vi "Handle Data Change.vi"(4 "Value":string, 6 "Combo Box Ref":refnum<vi>, 7 "Data in":path, 8 "error in (no error)":errorcluster, 9 "Run Mode?":bool, 10 "Indicator?":bool, 11 "Path Selector in":refnum<class "MGI Path Selector.lvclass">) -> (0 "error out":errorcluster, 3 "Path Selector out":refnum<class "MGI Path Selector.lvclass">, 5 "Data out":path)   [LabVIEW 2020, in "MGI Path Selector.lvclass"]
doc: "Take an action appropriate for the specified value of the combo box.\n\nAuthored by Shawn Walpole\nsupport@mooregoodideas.com\nwww.mooregoodideas.com\n\nCopyright (c) 2013, Moore Good Ideas, Inc.\n\nAll rights reserved.\n\nRedistribution and use in source and binary forms, with or without modification, are permitted provided that the following conditions are met:\n\n * Redistributions of source code must retain the above copyright notice, this list of conditions and the following disclaimer.\n * Redistributions in binary form must reproduce the above copyright notice, this list of conditions and the following disclaimer in the documentation and/or other materials provided with the distribution.\n * Neither the name of Moore Good Ideas, Inc. nor the names of its contributors may be used to endorse or promote products derived from this software without specific prior written permission.\n\nTHIS SOFTWARE IS PROVIDED BY THE COPYRIGHT HOLDERS AND CONTRIBUTORS \"AS IS\" AND ANY EXPRESS OR IMPLIED WARRANTIES, INCLUDING, BUT NOT LIMITED TO, THE IMPLIED WARRANTIES OF MERCHANTABILITY AND FITNESS FOR A PARTICULAR PURPOSE ARE DISCLAIMED. IN NO EVENT SHALL THE COPYRIGHT OWNER OR CONTRIBUTORS BE LIABLE FOR ANY DIRECT, INDIRECT, INCIDENTAL, SPECIAL, EXEMPLARY, OR CONSEQUENTIAL DAMAGES (INCLUDING, BUT NOT LIMITED TO, PROCUREMENT OF SUBSTITUTE GOODS OR SERVICES; LOSS OF USE, DATA, OR PROFITS; OR BUSINESS INTERRUPTION) HOWEVER CAUSED AND ON ANY THEORY OF LIABILITY, WHETHER IN CONTRACT, STRICT LIABILITY, OR TORT (INCLUDING NEGLIGENCE OR OTHERWISE) ARISING IN ANY WAY OUT OF THE USE OF THIS SOFTWARE, EVEN IF ADVISED OF THE POSSIBILITY OF SUCH DAMAGE."
uses:
  <userlib>/_MGI/User Interface/Path Selector XControl/Class Hierarchy/MGI Path Selector.lvclass
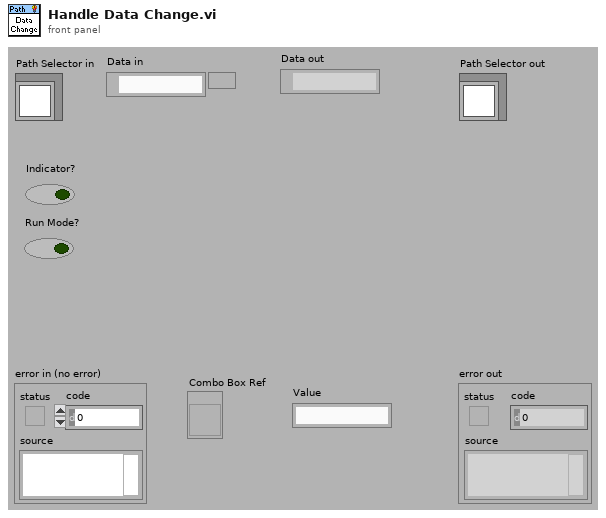
[diagram p1: front panel]
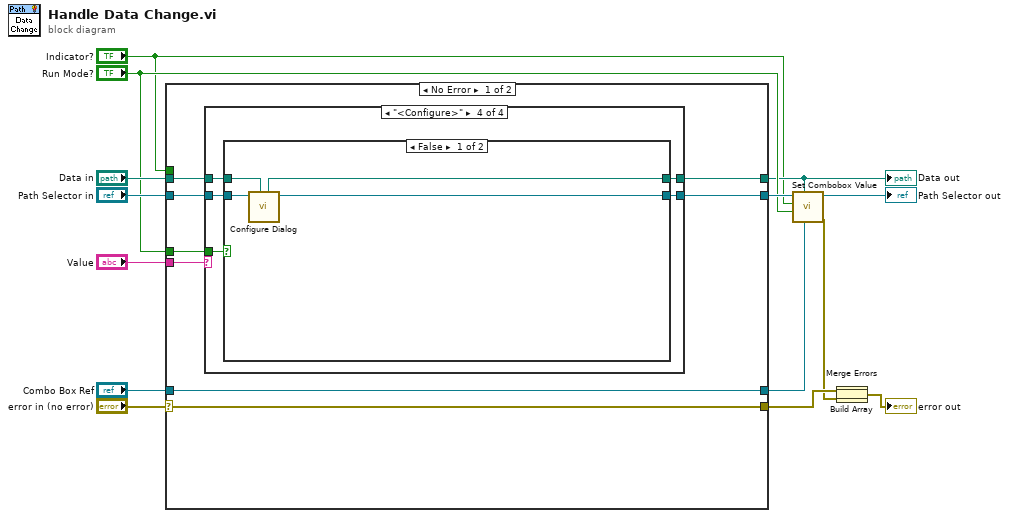
[diagram p0: block diagram]
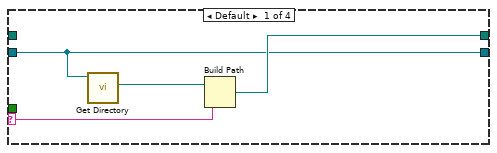
[diagram p2: hidden frame]
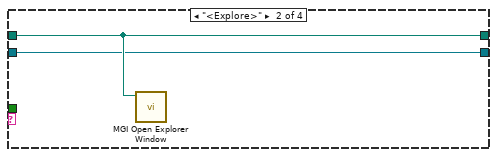
[diagram p3: hidden frame]
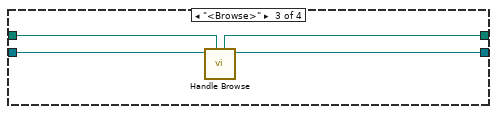
[diagram p4: hidden frame]
diagram:
  n1 = case shown="No Error" "error in (no error)" {
    selector: "error in (no error)" -> [w23 w48]
    tunnel: [w23 w48] -> w4
    tunnel: [w18 w47] -> w11
    tunnel: "Path Selector in" -> [w21 w47]
    tunnel: "Run Mode?" -> [w17 _]
    tunnel: "Combo Box Ref" -> [w16 w46]
    tunnel: "Value" -> [w22 _]
    tunnel: [w16 w46] -> w10
    tunnel: "Data in" -> [w20 w45]
    tunnel: [w19 w45] -> w7
    tunnel: "Indicator?" -> [_ _]
    frame No Error {
      n2 = case shown="\"<Configure>\"" w22 {
        selector: w22 -> [w26 _ _ _]
        tunnel: w20 -> [_ w29 w33 w36]
        tunnel: [w25 w29 w32 w35] -> w19
        tunnel: w21 -> [w24 w28 w30 w37]
        tunnel: [w24 w28 w31 w34] -> w18
        tunnel: w17 -> [_ _ _ w38]
        frame Default {
          n3 = call-dynamic "Get Directory.vi"("Path Selector in"=w24) -> ("Start Path"=w27:path)  [unwired: 9 in, 1 out]
          n4 = Build Path(base path=w27, name or relative path=w26) -> (appended path=w25:path)
        }
        frame "<Explore>" {
          n5 = call <userlib>:"MGI Open Explorer Window.vi"("Directory or File"=w29) -> ()  [unwired: 10 in, 1 out]
        }
        frame "<Browse>" {
          n6 = call-dynamic "Handle Browse.vi"("Data in"=w33, "Path Selector in"=w30) -> ("Path Selector out"=w31:refnum<class "MGI Path Selector.lvclass">, "Data out"=w32:path)  [unwired: 7 in, 1 out]
        }
        frame "<Configure>" {
          n7 = case shown="False" w38 {
            tunnel: w37 -> [w42 w43]
            tunnel: w36 -> [w39 w44]
            tunnel: [w40 w44] -> w35
            tunnel: [w41 w43] -> w34
            frame False {
              n8 = call-dynamic "Configure Dialog.vi"("Data in"=w39, "Path Selector in"=w42) -> ("Path Selector out"=w41:refnum<class "MGI Path Selector.lvclass">, "Data out"=w40:path)  [unwired: 7 in, 1 out]
            }
            frame True {
              # "Don't allow configure in run mode."
            }
          }
        }
      }
    }
    frame Error {
    }
  }
  "Data out" <- w7
  n9 = call-dynamic "Set Combobox Value.vi"("Combo Box Ref"=w10, "Data"=w7, "Run Mode?"="Run Mode?", "Indicator?"="Indicator?", "Path Selector in"=w11) -> ("error out"=w3:errorcluster, "Path Selector out"=→"Path Selector out":refnum<class "MGI Path Selector.lvclass">)  [unwired: 5 in]
  n10 = Build Array(w4, w3) -> (w1:errorcluster[])
  n11 = Merge Errors(w1) -> (→"error out":errorcluster)
